vi "BGA244_meas_purity.vi"(8 "error in":errorcluster, 11 "VISA in":refnum<visa-resource-name>) -> (0 "error out":errorcluster, 2 "purity":dbl, 3 "VISA out":refnum<visa-resource-name>, 4 "status":bool)   [LabVIEW 2019]
panel:
  out "string":string
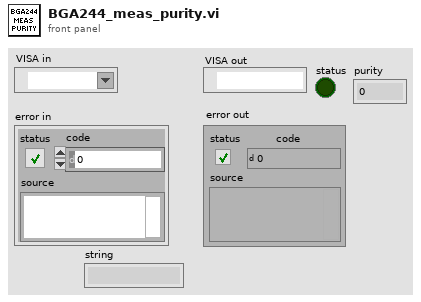
[diagram p1: front panel]
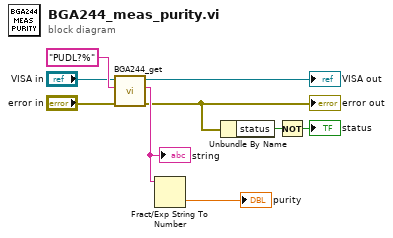
[diagram p0: block diagram]
diagram:
  n1 = call "BGA244_get.vi"("error in"="error in", "string in"="PUDL?%" ("string"), "VISA in"="VISA in") -> ("error out"=w3:errorcluster, "string out"=w5:string, "VISA out"=→"VISA out":refnum<visa-resource-name>)  [unwired: 6 in]
  "error out" <- w3
  "string" <- w5
  n2 = Fract/Exp String To Number(string=w5) -> (number=→"purity":dbl)  [unwired: 3 in, 1 out]
  n3 = Unbundle By Name(w3) -> ("status"=w2:bool)
  n4 = Not(x=w2) -> (.not. x?=→"status":bool)
